vi "Remove Handler(by Ref).vi"(8 "error in (no error)":errorcluster, 10 "Handler":refnum<class "Handler.lvclass">) -> (0 "error out":errorcluster)   [LabVIEW 2017, in "Error Log.lvlib" / "Logger.lvclass"]
doc: "Removes a handler specified by <b>Name</b> from the referenced ``*Logger``.. \nIf there is no handler with the searched name, nothing is removed and the error \"5030 - Item not found\" is returned."
uses:
  Logger.lvclass
  Handler/Handler.lvclass
  Logger.lvclass/Logger.ctl
  Handler/Handler.lvclass/Handler.ctl
  Set Handlers.vi
  Get Handlers.vi
  Handler/Get Name.vi
  Get Handler Names.vi
  <vilib>/Utility/error.llb/Error Cluster From Error Code.vi
  <vilib>/ErrorRing/Error Ring.xnode
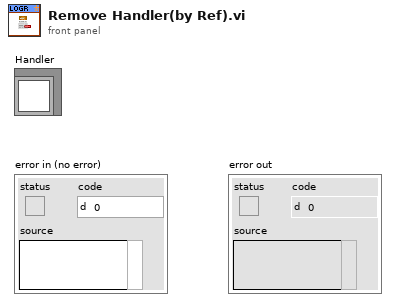
[diagram p1: front panel]
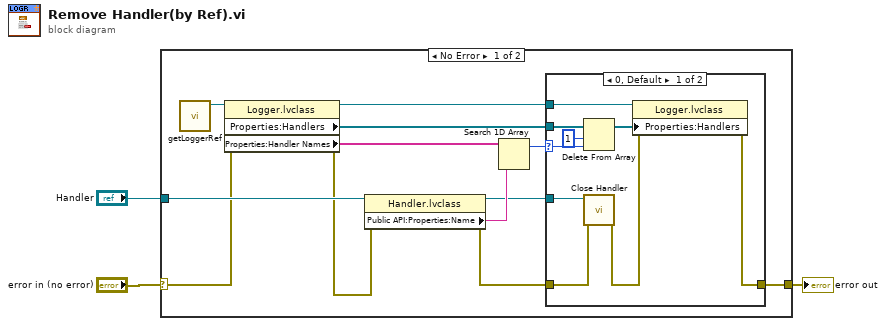
[diagram p0: block diagram]
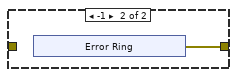
[diagram p2: hidden frame]
diagram:
  n1 = case shown="No Error" "error in (no error)" {
    selector: "error in (no error)" -> [w12 w31]
    tunnel: [w6 w31] -> w2
    tunnel: "Handler" -> [w15 _]
    frame No Error {
      n2 = call "getLoggerRef.vi"() -> ("Logger Ref"=w4:refnum<data-value>)  [unwired: 10 in, 1 out]
      n3 = property class="Logger.lvclass"(reference=w4, error in=w12) -> (reference out=w8:refnum<data-value>, error out=w11:errorcluster, "Properties:Handlers"=w10:refnum<class "Handler.lvclass">[], "Properties:Handler Names"=w14:string[])
      n4 = property class="Handler.lvclass"(reference=w15, error in=w11) -> (reference out=w5:refnum<class "Handler.lvclass">, error out=w7:errorcluster, "Public API:Properties:Name"=w13:string)
      n5 = Search 1D Array(1D array=w14, element=w13) -> (index of element=w9:i32)  [unwired: 1 in]
      n6 = case shown="0, Default" w9 {
        selector: w9 -> [w23 _]
        tunnel: w10 -> [w24 _]
        tunnel: w8 -> [w19 _]
        tunnel: w7 -> [w20 _]
        tunnel: [w16 w25] -> w6
        tunnel: w5 -> [w21 _]
        frame 0, Default {
          n7 = Delete From Array(array=w24, length=1, index=w23) -> (array with subset deleted=w18:refnum<class "Handler.lvclass">[])  [unwired: 1 out]
          n8 = call "Close Handler.vi"("error in (no error)"=w20, "Handler in"=w21) -> ("error out"=w17:errorcluster)  [unwired: 8 in, 1 out]
          n9 = property class="Logger.lvclass"(reference=w19, error in=w17, "Properties:Handlers"=w18) -> (error out=w16:errorcluster)  [unwired: 1 out]
        }
        frame -1 {
          n10 = xnode "Error Ring"() -> ("error out"=w25:errorcluster)
        }
      }
    }
    frame Error {
    }
  }
  "error out" <- w2
